vi "Sawtooth Wave.vi"(0 "samples":i32=128, 1 "amplitude":dbl=1.0 format="%0.2f", 2 "f":dbl=0.0078125 format="%0.4e", 3 "phase in":dbl format="%0.2f", 4 "reset phase":bool=TRUE) -> (5 "sawtooth wave":dbl[](array[numeric]) format="%0.2f", 6 "phase out":dbl format="%0.2e", 7 "error":i32)   [LabVIEW 2009]
doc: "Generates an array containing a sawtooth wave."
uses:
  C:/Program Files/National Instruments/LabVIEW 2009/resource/lvanlys.dll
panel:
  # "Sawtooth Wave"
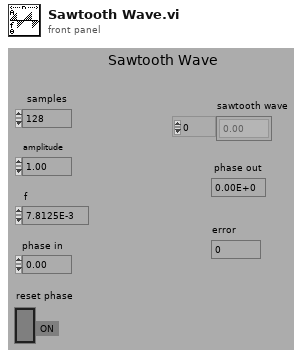
[diagram p1: front panel]
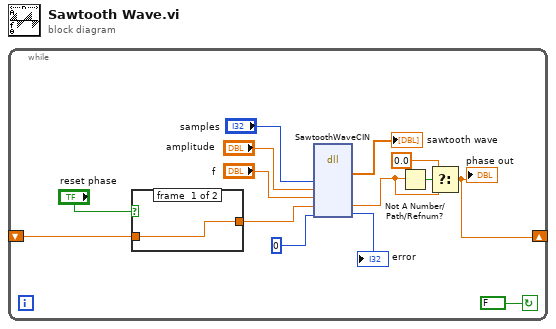
[diagram p0: block diagram]
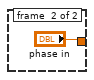
[diagram p2: hidden frame]
diagram:
  n1 = while {
    shift-left: _ -> [w14]
    shift-right: [w10] -> _
    stop <- FALSE continue-if-true
    n2 = case shown="True" "reset phase" {
      tunnel: [w15 "phase in"] -> w7
      tunnel: w14 -> [w15 _]
      frame #0 {
      }
      frame #1 {
      }
    }
    n3 = dll-call lib="C:/Program Files/National Instruments/LabVIEW 2009/resource/lvanlys.*" fn="SawtoothWaveCIN"("samples"="samples", "amplitude"="amplitude", "f"="f", "phase in"=w7, 0) -> ("sawtooth wave"=→"sawtooth wave":dbl[], "phase in"=w6:dbl, →"error":i32)  [unwired: 8 in, 2 out]
    n4 = Not A Number/Path/Refnum?(number/path/refnum=w6) -> (NaN/Path/Refnum?=w12:bool)
    n5 = Select(t=0.0, s=w12, f=w6) -> (s? t:f=w10:dbl)
    "phase out" <- w10
  }
